vi "R1DOControl_Status.vi"(7 "LabVIEW Web Service Request":refnum<class "Web Request.lvclass">) -> (3 "DOData":T1 {"DO_Manual"."N2 MFC" scale=0.0..500.0; "DO_Manual"."Air MFC" scale=0.0..500.0})   [LabVIEW 2016]
uses:
  R1Controls/R7DO_Status.ctl
  <vilib>/wsapi/Web Request.lvclass
panel:
  # "Use the Web Service Request input terminal to call the VIs on the Web Services palette. Do not remove it from the connector pane unless you don't need access to the palette."
  # "Each additional control wired to the connector pane will be available as an input in the URL. To include an indicator in terminal-mode output (the default setting), it must also be wired to the connector pane."
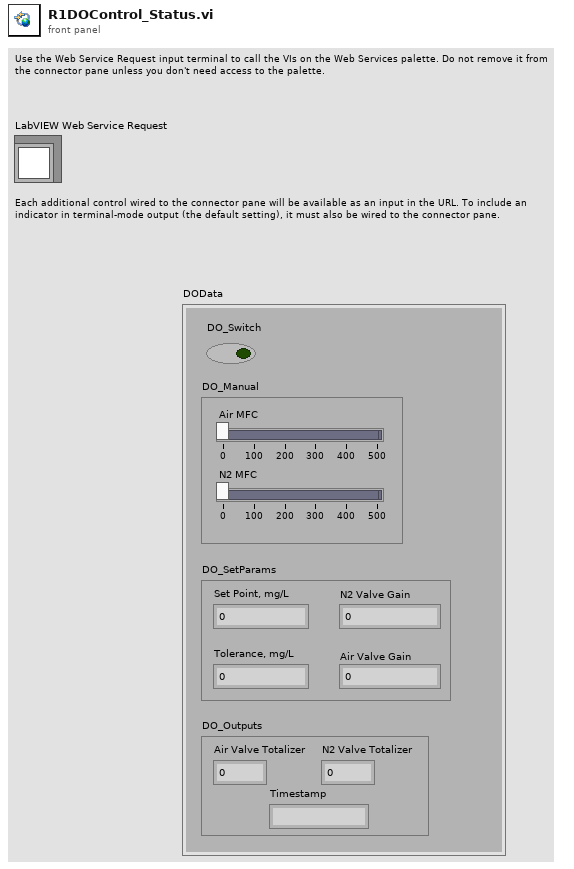
[diagram p1: front panel]
types:
  T1 = typedef "R7DO_Status.ctl" = cluster{"DO_Switch":bool, "DO_Manual":cluster{"Air MFC":dbl, "N2 MFC":dbl}, "DO_Outputs":cluster{"Timestamp":string, "Air Valve Totalizer":dbl, "N2 Valve Totalizer":dbl}, "DO_SetParams":cluster{"Set Point, mg/L":dbl, "Tolerance, mg/L":dbl, "N2 Valve Gain":dbl, "Air Valve Gain":dbl}}
  T2 = cluster{"Set Point, mg/L":dbl, "Tolerance, mg/L":dbl, "N2 Valve Gain":dbl, "Air Valve Gain":dbl}
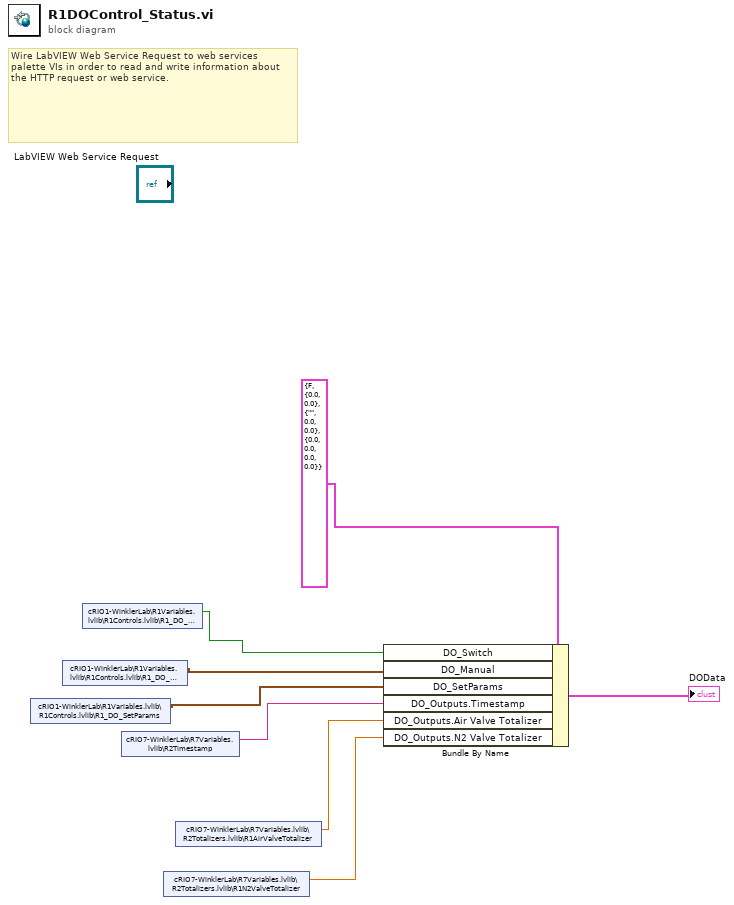
[diagram p0: block diagram]
diagram:
  # "Wire LabVIEW Web Service Request to web services palette VIs in order to read and write information about the HTTP request or web service."
  n1 = shared-variable "cRIO1-WinklerLab\\R1Variables.lvlib\\R1Controls.lvlib\\R1_DO_SetParams"() -> (w5:T2)  [unwired: 1 in, 1 out]
  n2 = shared-variable "cRIO1-WinklerLab\\R1Variables.lvlib\\R1Controls.lvlib\\R1_DO_Manual"() -> (w4:cluster{"Air MFC":dbl, "N2 MFC":dbl})  [unwired: 1 in, 1 out]
  n3 = shared-variable "cRIO1-WinklerLab\\R1Variables.lvlib\\R1Controls.lvlib\\R1_DO_Switch"() -> (w6:bool)  [unwired: 1 in, 1 out]
  n4 = shared-variable "cRIO7-WinklerLab\\R7Variables.lvlib\\R2Timestamp"() -> (w8:string)  [unwired: 1 in, 1 out]
  n5 = shared-variable "cRIO7-WinklerLab\\R7Variables.lvlib\\R2Totalizers.lvlib\\R1N2ValveTotalizer"() -> (w1:dbl)  [unwired: 1 in, 1 out]
  n6 = shared-variable "cRIO7-WinklerLab\\R7Variables.lvlib\\R2Totalizers.lvlib\\R1AirValveTotalizer"() -> (w2:dbl)  [unwired: 1 in, 1 out]
  n7 = Bundle By Name(cluster=T1 {"DO_Switch"=FALSE, "DO_Manual"={"Air MFC"=0.0, "N2 MFC"=0.0}, "DO_Outputs"={"Timestamp"="", "Air Valve Totalizer"=0.0, "N2 Valve Totalizer"=0.0}, "DO_SetParams"={"Set Point, mg/L"=0.0, "Tolerance, mg/L"=0.0, "N2 Valve Gain"=0.0, "Air Valve Gain"=0.0}} ("DOData"), "DO_Switch"=w6, "DO_Manual"=w4, "DO_SetParams"=w5, "DO_Outputs.Timestamp"=w8, "DO_Outputs.Air Valve Totalizer"=w2, "DO_Outputs.N2 Valve Totalizer"=w1) -> (→"DOData":T1)
